vi "CI_CapacityState.vi"(0 "Display State In":T2={"StandardColor"=6881066, "WarningColor"=16766208, "CriticalColor"=15671808, "Standard<>Warning Range"=75, "Warning<>Critical Range"=95}, 9 "Container State":T3, 11 "error in (no error)":errorcluster) -> (4 "Display State Out":T2={"StandardColor"=6881066, "WarningColor"=16766208, "CriticalColor"=15671808, "Standard<>Warning Range"=75, "Warning<>Critical Range"=95}, 6 "CapacityStates":T1, 15 "error out":errorcluster)   [LabVIEW 2010, in "CapacityIndicator.xctl"]
doc: "Get the actual capacity state."
uses:
  CapacityIndicator.xctl
  <vilib>/_xctls/Container State.ctl
  CI_State.ctl
  VIs/CI_CapacityStates.ctl
  <vilib>/_xctls/XControlSupport.lvlib
panel:
  # "Add Controls & Indicators that form the parameters of the method here. Hook them to the connector pane. Do not delete the controls & indicators that are already hooked to the connector pane.\n \nTo setup the parameters  for this method, right click on this item in the Project Tree & select \"Configure Method...\"."
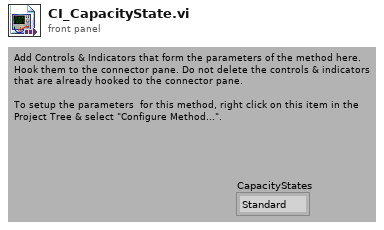
[diagram p1: front panel]
types:
  T1 = typedef "CapacityIndicator.xctl/CI_CapacityStates.ctl" = enum16{"Standard", "Warning", "Critical"}
  T2 = typedef "CapacityIndicator.xctl/CI_State.ctl" = cluster{"StandardColor":u32, "WarningColor":u32, "CriticalColor":u32, "Standard<>Warning Range":u8, "Warning<>Critical Range":u8}
  T3 = typedef "XControlSupport.lvlib/Container State.ctl" = cluster{"Indicator?":bool, "Run Mode?":bool, " Refnum":refnum<vi>}
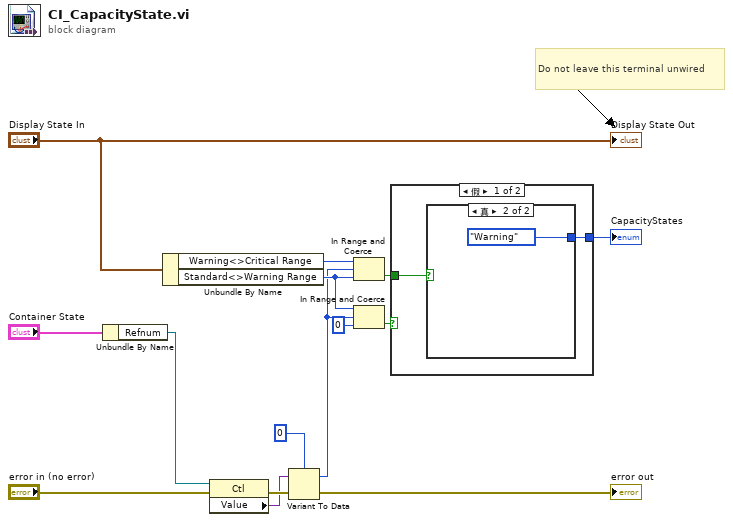
[diagram p0: block diagram]
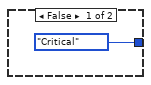
[diagram p2: hidden frame]
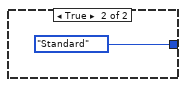
[diagram p3: hidden frame]
diagram:
  # "Do not leave this terminal unwired"
  n1 = Unbundle By Name("Container State") -> ("Refnum"=w14:refnum<vi>)
  n2 = Unbundle By Name("Display State In") -> ("Warning<>Critical Range"=w6:u8, "Standard<>Warning Range"=w7:u8)
  n3 = property class="Ctl"(reference=w14, error in="error in (no error)") -> (error out=w12:errorcluster, "Value"=w9:variant)  [unwired: 1 out]
  n4 = Variant To Data(error in=w12, Variant=w9, type=u8 0) -> (error out=→"error out":errorcluster, data=w3:u8)
  n5 = In Range and Coerce(upper limit=w6, x=w3, lower limit=w7) -> (In Range?=w4:bool)  [unwired: 1 out]
  n6 = In Range and Coerce(upper limit=w7, x=w3, lower limit=u8 0) -> (In Range?=w5:bool)  [unwired: 1 out]
  n7 = case shown="假" w5 {
    tunnel: w4 -> [w16 _]
    tunnel: [w17 CI_CapacityStates."Standard" ("CapacityStates")] -> w1
    frame False {
      n8 = case shown="真" w16 {
        tunnel: [CI_CapacityStates."Critical" ("CapacityStates") CI_CapacityStates."Warning" ("CapacityStates")] -> w17
        frame False {
        }
        frame True {
        }
      }
    }
    frame True {
    }
  }
  "CapacityStates" <- w1
  "Display State Out" <- "Display State In"
